vi "Odour_drag.vi"(9 "Data":T1(array[cluster]), 10 "Array in":string[](array[string]), 11 "Odour chemicals":T2(array[cluster])) -> (2 "Boolean":bool, 3 "Array out":T1(array[cluster]))   [LabVIEW 2016]
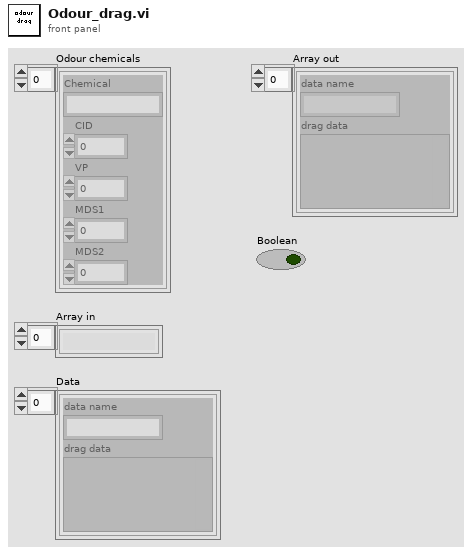
[diagram p1: front panel]
types:
  T1 = cluster{"data name":string, "drag data":variant}[]
  T2 = cluster{"Chemical":string, "CID":i32, "VP":dbl, "MDS1":dbl, "MDS2":dbl}[]
  T3 = cluster{"Chemical":string, "CID":i32, "VP":dbl, "MDS1":dbl, "MDS2":dbl}
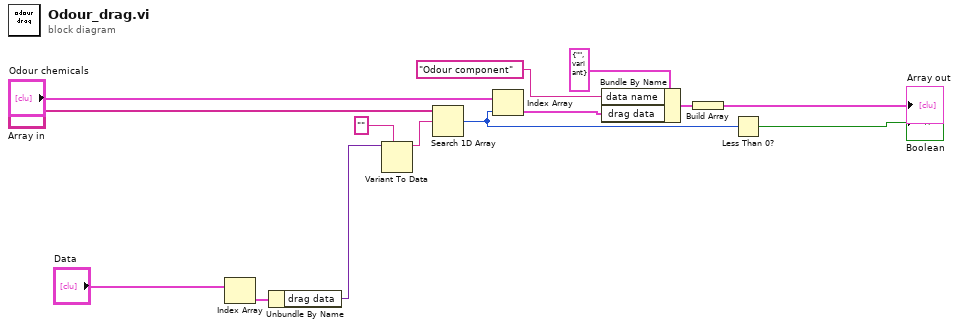
[diagram p0: block diagram]
diagram:
  n1 = Index Array(array="Data") -> (element=w2:cluster{"data name":string, "drag data":variant})  [unwired: 1 in]
  n2 = Unbundle By Name(w2) -> ("drag data"=w3:variant)
  n3 = Variant To Data(type="", Variant=w3) -> (data=w6:string)  [unwired: 1 in, 1 out]
  n4 = Search 1D Array(1D array="Array in", element=w6) -> (index of element=w11:i32)  [unwired: 1 in]
  n5 = Index Array(array="Odour chemicals", index=w11) -> (element=w12:T3)
  n6 = Bundle By Name(cluster=cluster{"data name":string, "drag data":variant} {"data name"="", "drag data"=variant}, "data name"="Odour component", "drag data"=w12) -> (w13:cluster{"data name":string, "drag data":variant})
  n7 = Build Array(w13) -> (→"Array out":T1)
  n8 = Less Than 0?(x=w11) -> (x < 0?=→"Boolean":bool)
